vi "Check Limits.vi"(8 "error in (no error)":errorcluster, 11 "System Health Module in":refnum<class "System Health Module.lvclass">) -> (0 "error out":errorcluster, 3 "System Health Module out":refnum<class "System Health Module.lvclass">)   [LabVIEW 2020, in "Volatus.lvlib" / "System Health Module.lvclass"]
uses:
  System Health Module.lvclass
  System Health Module.lvclass/System Health Module.ctl
  Module/Module.lvclass
  Event Level.ctl
  Volatus.lvlib
  System SAL/System SAL.lvclass
  C:/dev/lv20CE/relink/lv-volatus/Volatus/Module/Module.lvclass
  C:/dev/lv20CE/relink/lv-volatus/Volatus/System Health Module/System Health Module.lvclass
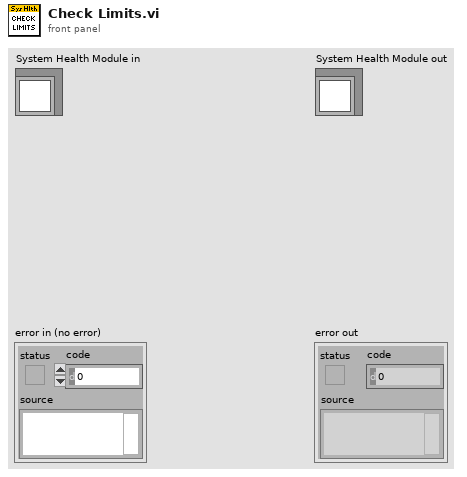
[diagram p1: front panel]
types:
  T1 = typedef "Volatus.lvlib/System Health Module.lvclass/Drive Info.ctl" = cluster{"Config":T2, "Capacity GB":dbl, "Used GB":dbl, "Next Warning":dbl, "Next Error":dbl}
  T2 = typedef "Volatus.lvlib/System Health Module.lvclass/Drive Config.ctl" = cluster{"Path":path, "Warning GB":dbl, "Error GB":dbl}
  T3 = typedef "Volatus.lvlib/Event Level.ctl" = enum16{"Debug", "Info", "Warning", "Error"}
  T4 = typedef "Volatus.lvlib/System SAL.lvclass/Performance Values.ctl" = cluster{"CPU Total %":dbl, "Mem Avail GB":dbl, "Mem Free GB":dbl}
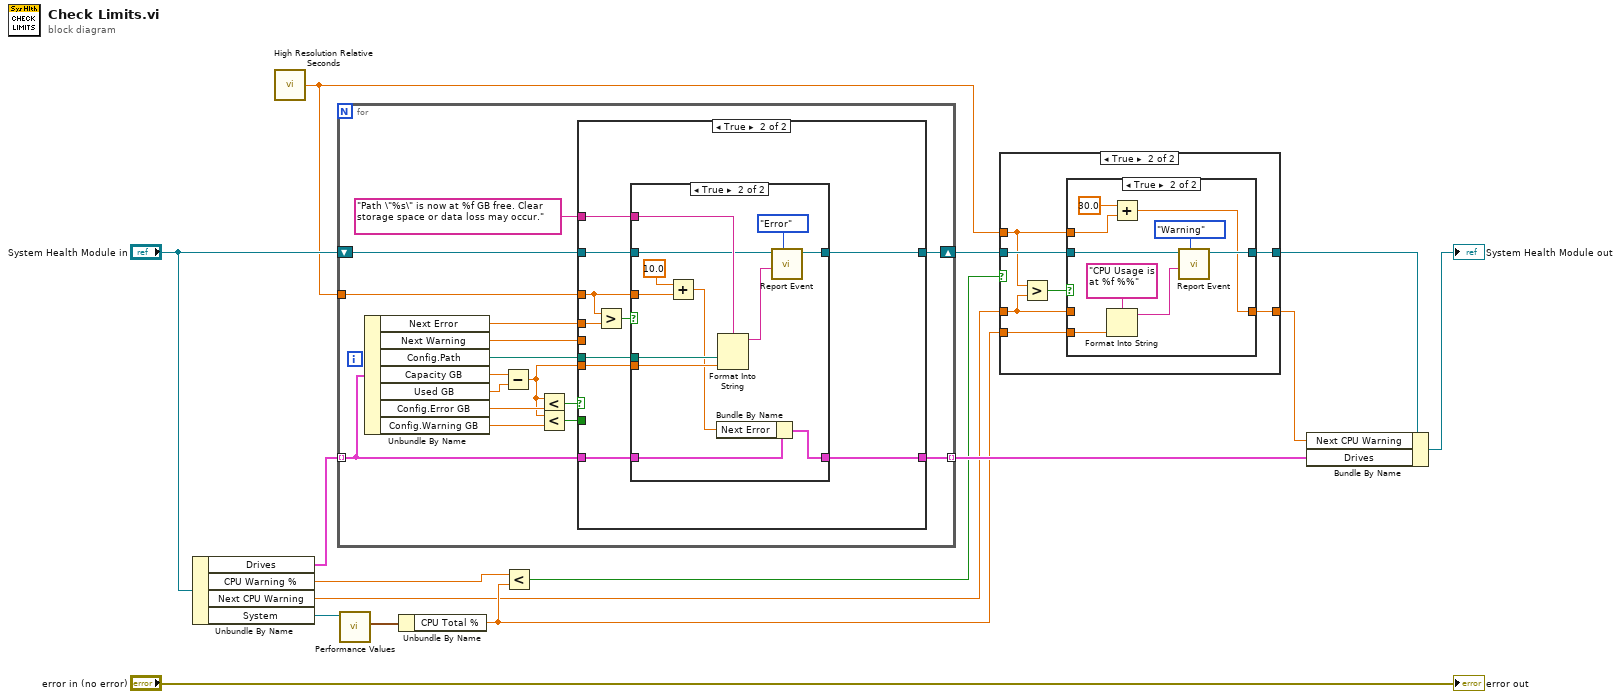
[diagram p0: block diagram]
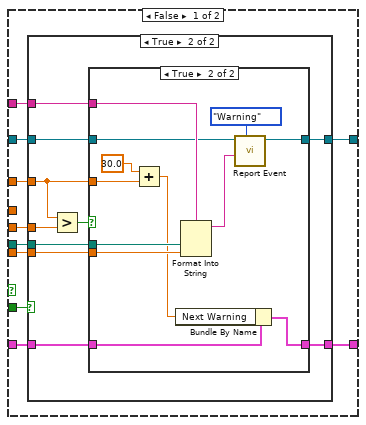
[diagram p4: hidden frame]
diagram:
  n1 = Unbundle By Name("System Health Module in") -> ("Drives"=w14:T1[], "CPU Warning %"=w8:dbl, "Next CPU Warning"=w3:dbl, "System"=w12:refnum<class "System SAL.lvclass">)
  n2 = call <vilib>:"High Resolution Relative Seconds.vi"() -> ("relative seconds"=w2:dbl)
  n3 = for {
    tunnel: w14 -> [w19] mode=indexing
    shift-right: [w22] -> w7
    shift-left: "System Health Module in" -> [w23]
    tunnel: w2 -> [w20]
    tunnel: [w17] -> w9 mode=indexing
    n4 = Unbundle By Name(w19) -> ("Next Error"=w21:dbl, "Next Warning"=w16:dbl, "Config.Path"=w28:path, "Capacity GB"=w31:dbl, "Used GB"=w30:dbl, "Config.Error GB"=w27:dbl, "Config.Warning GB"=w26:dbl)
    n5 = Subtract(x=w31, y=w30) -> (x-y=w25:dbl)
    n6 = Less?(x=w25, y=w27) -> (x < y?=w29:bool)
    n7 = Less?(x=w25, y=w26) -> (x < y?=w24:bool)
    n8 = case shown="True" w29 {
      tunnel: w28 -> [w39 w76]
      tunnel: "Path \"%s\" is now at %f GB free. Clear storage space or data loss may occur." -> [w38 w77]
      tunnel: w25 -> [w40 w75]
      tunnel: w24 -> [w41 _]
      tunnel: w23 -> [w37 w74]
      tunnel: [w36 w73] -> w22
      tunnel: w21 -> [_ w72]
      tunnel: w20 -> [w35 w70]
      tunnel: w19 -> [w34 w69]
      tunnel: [w33 w68] -> w17
      tunnel: w16 -> [w32 _]
      frame False {
        n9 = case shown="True" w41 {
          tunnel: w40 -> [_ w51]
          tunnel: w39 -> [_ w52]
          tunnel: w38 -> [_ w53]
          tunnel: w37 -> [w43 w50]
          tunnel: [w43 w49] -> w36
          tunnel: w35 -> [_ w45]
          tunnel: w34 -> [w42 w48]
          tunnel: [w42 w47] -> w33
          tunnel: w32 -> [_ w46]
          frame False {
          }
          frame True {
            n10 = Greater?(x=w45, y=w46) -> (0:w44:bool)
            n11 = case shown="True" w44 {
              tunnel: w53 -> [_ w67]
              tunnel: w52 -> [_ w66]
              tunnel: w51 -> [_ w65]
              tunnel: w50 -> [w55 w64]
              tunnel: [w55 w62] -> w49
              tunnel: w45 -> [_ w60]
              tunnel: w48 -> [w54 w58]
              tunnel: [w54 w56] -> w47
              frame False {
              }
              frame True {
                n12 = Add(x=30.0, y=w60) -> (x+y=w57:dbl)
                n13 = Bundle By Name(cluster=w58, "Next Warning"=w57) -> (w56:T1)
                n14 = Format Into String(format string=w67, w66, w65) -> (resulting string=w61:string)  [unwired: 2 in, 1 out]
                n15 = call "Report Event.vi"("Level (Info)"=Event_Level."Warning", "Message"=w61, "Module in"=w64) -> ("Module out"=w62:refnum<class "System Health Module.lvclass">)  [unwired: 7 in, 1 out]
              }
            }
          }
        }
      }
      frame True {
        n16 = Greater?(x=w70, y=w72) -> (0:w71:bool)
        n17 = case shown="True" w71 {
          tunnel: w77 -> [_ w91]
          tunnel: w76 -> [_ w90]
          tunnel: w75 -> [_ w89]
          tunnel: w74 -> [w78 w87]
          tunnel: [w78 w85] -> w73
          tunnel: w70 -> [_ w84]
          tunnel: w69 -> [w79 w82]
          tunnel: [w79 w80] -> w68
          frame False {
          }
          frame True {
            n18 = Add(x=10.0, y=w84) -> (x+y=w81:dbl)
            n19 = Bundle By Name(cluster=w82, "Next Error"=w81) -> (w80:T1)
            n20 = Format Into String(format string=w91, w90, w89) -> (resulting string=w86:string)  [unwired: 2 in, 1 out]
            n21 = call "Report Event.vi"("Level (Info)"=Event_Level."Error", "Message"=w86, "Module in"=w87) -> ("Module out"=w85:refnum<class "System Health Module.lvclass">)  [unwired: 7 in, 1 out]
          }
        }
      }
    }
  }
  n22 = call-dynamic "Performance Values.vi"("System SAL in"=w12) -> ("Performance Values"=w11:T4)  [unwired: 9 in, 1 out]
  n23 = Unbundle By Name(w11) -> ("CPU Total %"=w4:dbl)
  n24 = Less?(x=w8, y=w4) -> (x < y?=w5:bool)
  n25 = case shown="True" w5 {
    tunnel: w7 -> [w92 w100]
    tunnel: [w92 w99] -> w6
    tunnel: w4 -> [_ w98]
    tunnel: w3 -> [w93 w95]
    tunnel: w2 -> [_ w96]
    tunnel: [w93 w94] -> w1
    frame False {
    }
    frame True {
      n26 = Greater?(x=w96, y=w95) -> (0:w97:bool)
      n27 = case shown="True" w97 {
        tunnel: w100 -> [w101 w110]
        tunnel: [w101 w109] -> w99
        tunnel: w98 -> [_ w106]
        tunnel: w96 -> [_ w108]
        tunnel: w95 -> [w102 _]
        tunnel: [w102 w103] -> w94
        frame False {
        }
        frame True {
          n28 = Format Into String(format string="CPU Usage is at %f %%", w106) -> (resulting string=w104:string)  [unwired: 2 in, 1 out]
          n29 = Add(x=30.0, y=w108) -> (x+y=w103:dbl)
          n30 = call "Report Event.vi"("Level (Info)"=Event_Level."Warning", "Message"=w104, "Module in"=w110) -> ("Module out"=w109:refnum<class "System Health Module.lvclass">)  [unwired: 7 in, 1 out]
        }
      }
    }
  }
  n31 = Bundle By Name(cluster=w6, "Next CPU Warning"=w1, "Drives"=w9) -> (→"System Health Module out":refnum<class "System Health Module.lvclass">)
  "error out" <- "error in (no error)"
